vi "getStatusReport.vi"(2 "device":string, 3 "ListRef":refnum<queue>) -> (0 "output report":string)   [LabVIEW 2012]
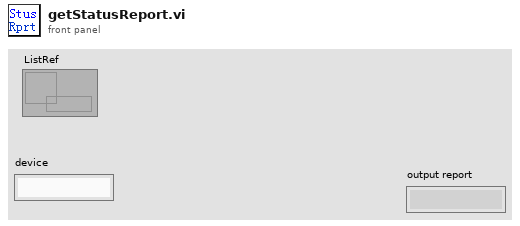
[diagram p1: front panel]
types:
  T1 = cluster{"DeviceID":string, "Channel":string, "param1":dbl, "Operation":string}
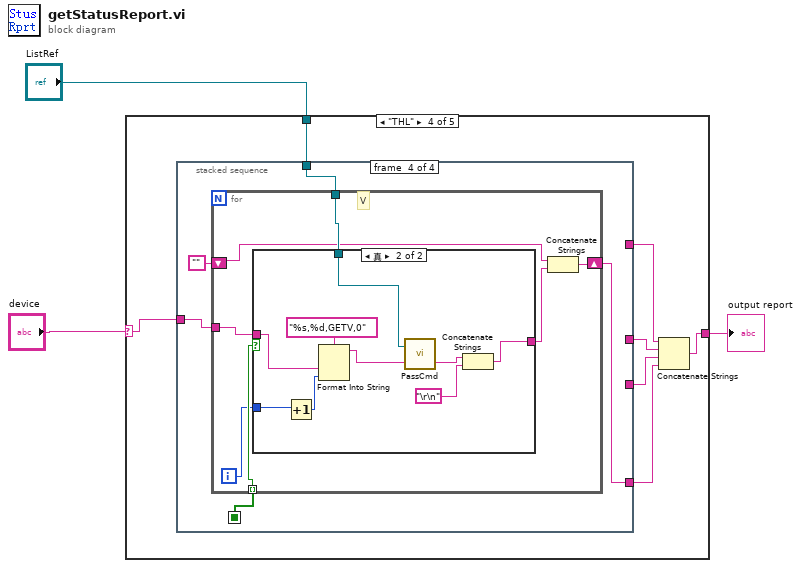
[diagram p0: block diagram]
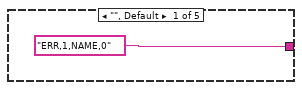
[diagram p2: hidden frame]
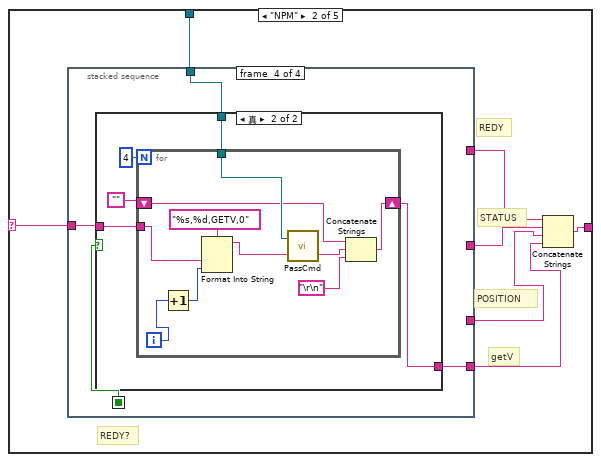
[diagram p3: hidden frame]
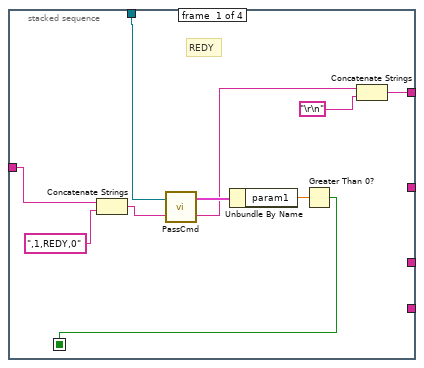
[diagram p4: hidden frame]
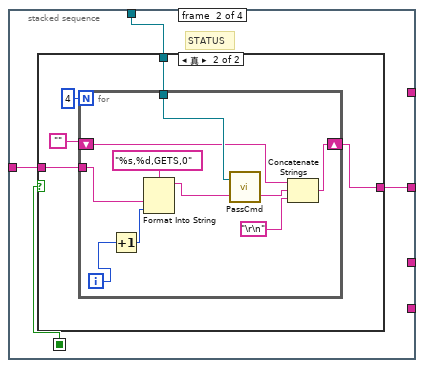
[diagram p5: hidden frame]
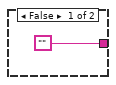
[diagram p6: hidden frame]
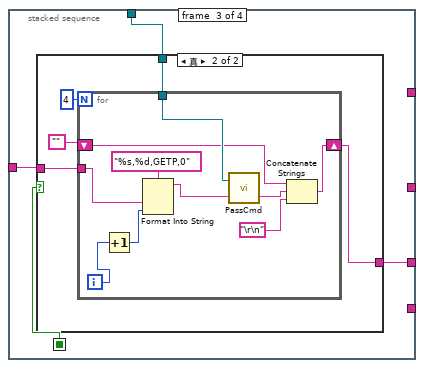
[diagram p7: hidden frame]
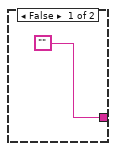
[diagram p8: hidden frame]
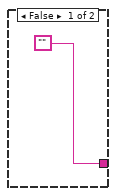
[diagram p9: hidden frame]
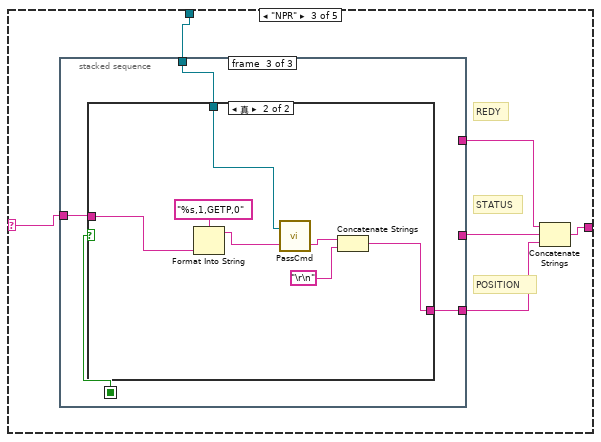
[diagram p10: hidden frame]
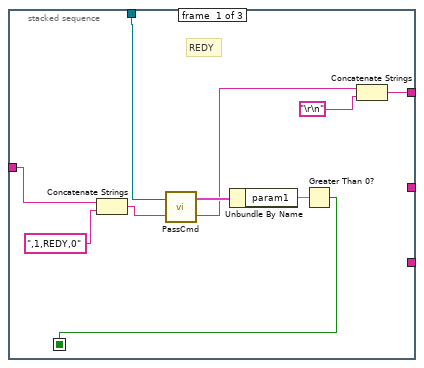
[diagram p11: hidden frame]
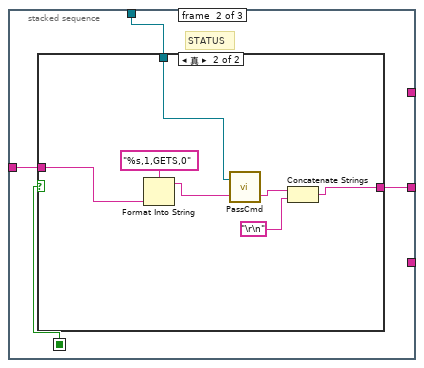
[diagram p12: hidden frame]
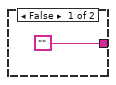
[diagram p13: hidden frame]
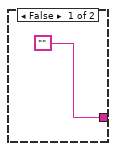
[diagram p14: hidden frame]
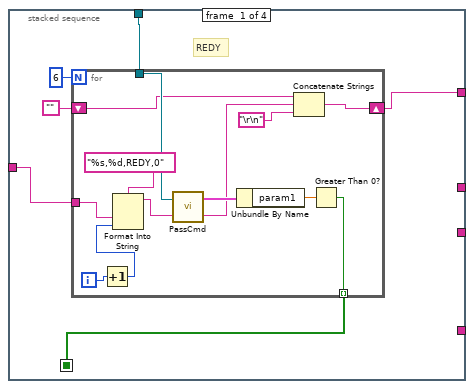
[diagram p15: hidden frame]
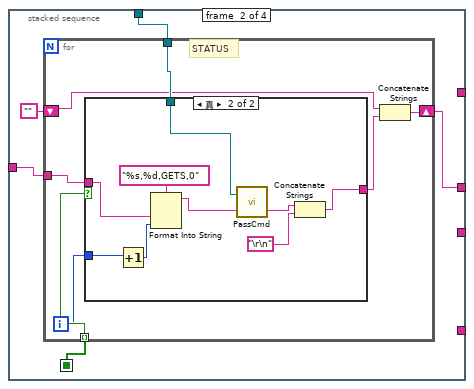
[diagram p16: hidden frame]
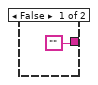
[diagram p17: hidden frame]
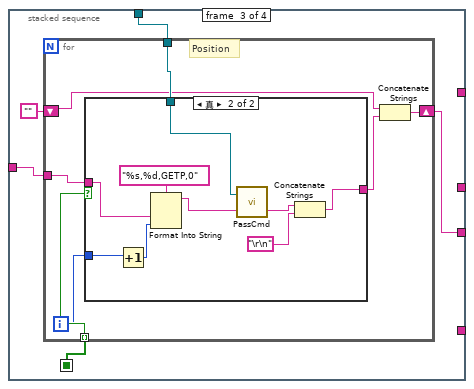
[diagram p18: hidden frame]
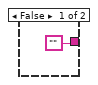
[diagram p19: hidden frame]
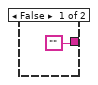
[diagram p20: hidden frame]
diagram:
  n1 = case shown="\"THL\"" "device" {
    selector: "device" -> [_ w11 w86 w127 w215]
    tunnel: ["ERR,1,NAME,0" w9 w82 w126 w214] -> w2
    tunnel: "ListRef" -> [_ w10 w87 w128 w216]
    frame "", Default {
    }
    frame "NPM" {
      # "getV"
      # "POSITION"
      # "STATUS"
      # "REDY"
      # "REDY?"
      n2 = stacked-sequence {
        seq-local: [w15 _ _ _] -> [_ w25 w45 w65]
        tunnel: w11 -> [w21 w24 w43 w63]
        tunnel: w10 -> [w18 w22 w44 w64]
        tunnel: [_ w23 _ _] -> w7
        tunnel: [w14 _ _ _] -> w8
        tunnel: [_ _ w42 _] -> w6
        tunnel: [_ _ _ w62] -> w5
        frame #0 {
          # "REDY"
          n3 = Concatenate Strings(w21, ",1,REDY,0") -> (w19:string)
          n4 = call "PassCmd.vi"("cmd in"=w19, "list ref"=w18) -> ("str out"=w13:string, "cmd out"=w17:T1)
          n5 = Unbundle By Name(w17) -> ("param1"=w16:dbl)
          n6 = Greater Than 0?(x=w16) -> (x > 0?=w15:bool)
          n7 = Concatenate Strings(w13, "\r\n") -> (w14:string)
        }
        frame #1 {
          # "STATUS"
          n8 = case shown="真" w25 {
            tunnel: w24 -> [_ w30]
            tunnel: ["" w27] -> w23
            tunnel: w22 -> [_ w29]
            frame False {
            }
            frame True {
              n9 = for {
                N: 4 -> [_]
                tunnel: w30 -> [w40]
                tunnel: w29 -> [w37]
                shift-right: [w33] -> w27
                shift-left: "" -> [w36]
                i -> [w32]
                n10 = Increment(x=w32) -> (x+1=w39:i32)
                n11 = Format Into String(format string="%s,%d,GETS,0" ("格式字符串"), w40, w39) -> (resulting string=w38:string)  [unwired: 2 in, 1 out]
                n12 = call "PassCmd.vi"("cmd in"=w38, "list ref"=w37) -> ("str out"=w35:string)  [unwired: 1 out]
                n13 = Concatenate Strings(w36, w35, "\r\n") -> (w33:string)
              }
            }
          }
        }
        frame #2 {
          n14 = case shown="真" w45 {
            tunnel: w43 -> [_ w50]
            tunnel: ["" w47] -> w42
            tunnel: w44 -> [_ w49]
            frame False {
            }
            frame True {
              n15 = for {
                N: 4 -> [_]
                tunnel: w50 -> [w60]
                tunnel: w49 -> [w57]
                shift-right: [w53] -> w47
                shift-left: "" -> [w56]
                i -> [w52]
                n16 = Increment(x=w52) -> (x+1=w59:i32)
                n17 = Format Into String(format string="%s,%d,GETP,0" ("格式字符串"), w60, w59) -> (resulting string=w58:string)  [unwired: 2 in, 1 out]
                n18 = call "PassCmd.vi"("cmd in"=w58, "list ref"=w57) -> ("str out"=w55:string)  [unwired: 1 out]
                n19 = Concatenate Strings(w56, w55, "\r\n") -> (w53:string)
              }
            }
          }
        }
        frame #3 {
          n20 = case shown="真" w65 {
            tunnel: w63 -> [_ w70]
            tunnel: ["" w67] -> w62
            tunnel: w64 -> [_ w69]
            frame False {
            }
            frame True {
              n21 = for {
                N: 4 -> [_]
                tunnel: w70 -> [w80]
                tunnel: w69 -> [w77]
                shift-right: [w73] -> w67
                shift-left: "" -> [w76]
                i -> [w72]
                n22 = Increment(x=w72) -> (x+1=w79:i32)
                n23 = Format Into String(format string="%s,%d,GETV,0" ("格式字符串"), w80, w79) -> (resulting string=w78:string)  [unwired: 2 in, 1 out]
                n24 = call "PassCmd.vi"("cmd in"=w78, "list ref"=w77) -> ("str out"=w75:string)  [unwired: 1 out]
                n25 = Concatenate Strings(w76, w75, "\r\n") -> (w73:string)
              }
            }
          }
        }
      }
      n26 = Concatenate Strings(w8, w7, w6, w5) -> (w9:string)
    }
    frame "NPR" {
      # "POSITION"
      # "STATUS"
      # "REDY"
      n27 = stacked-sequence {
        seq-local: [w91 _ _] -> [_ w101 w113]
        tunnel: w86 -> [w97 w100 w111]
        tunnel: w87 -> [w94 w98 w112]
        tunnel: [_ w99 _] -> w84
        tunnel: [w90 _ _] -> w85
        tunnel: [_ _ w110] -> w83
        frame #0 {
          # "REDY"
          n28 = Concatenate Strings(w97, ",1,REDY,0") -> (w95:string)
          n29 = call "PassCmd.vi"("cmd in"=w95, "list ref"=w94) -> ("str out"=w89:string, "cmd out"=w93:T1)
          n30 = Unbundle By Name(w93) -> ("param1"=w92:dbl)
          n31 = Greater Than 0?(x=w92) -> (x > 0?=w91:bool)
          n32 = Concatenate Strings(w89, "\r\n") -> (w90:string)
        }
        frame #1 {
          # "STATUS"
          n33 = case shown="真" w101 {
            tunnel: w100 -> [_ w109]
            tunnel: ["" w107] -> w99
            tunnel: w98 -> [_ w108]
            frame False {
            }
            frame True {
              n34 = Format Into String(format string="%s,1,GETS,0" ("格式字符串"), w109) -> (resulting string=w105:string)  [unwired: 2 in, 1 out]
              n35 = call "PassCmd.vi"("cmd in"=w105, "list ref"=w108) -> ("str out"=w104:string)  [unwired: 1 out]
              n36 = Concatenate Strings(w104, "\r\n") -> (w107:string)
            }
          }
        }
        frame #2 {
          n37 = case shown="真" w113 {
            tunnel: w111 -> [_ w121]
            tunnel: ["" w119] -> w110
            tunnel: w112 -> [_ w120]
            frame False {
            }
            frame True {
              n38 = Format Into String(format string="%s,1,GETP,0" ("格式字符串"), w121) -> (resulting string=w117:string)  [unwired: 2 in, 1 out]
              n39 = call "PassCmd.vi"("cmd in"=w117, "list ref"=w120) -> ("str out"=w116:string)  [unwired: 1 out]
              n40 = Concatenate Strings(w116, "\r\n") -> (w119:string)
            }
          }
        }
      }
      n41 = Concatenate Strings(w85, w84, w83) -> (w82:string)
    }
    frame "THL" {
      n42 = stacked-sequence {
        seq-local: [w132 _ _ _] -> [_ w149 w172 w194]
        tunnel: w127 -> [w134 w152 w174 w196]
        tunnel: w128 -> [w133 w150 w173 w195]
        tunnel: [_ w151 _ _] -> w124
        tunnel: [w131 _ _ _] -> w125
        tunnel: [_ _ w170 _] -> w123
        tunnel: [_ _ _ w192] -> w122
        frame #0 {
          # "REDY"
          n43 = for {
            N: 6 -> [_]
            tunnel: w134 -> [w137]
            tunnel: w133 -> [w147]
            tunnel: [w144] -> w132 mode=indexing
            shift-right: [w143] -> w131
            shift-left: "" -> [w136]
            i -> [w139]
            n44 = Increment(x=w139) -> (x+1=w138:i32)
            n45 = Format Into String(format string="%s,%d,REDY,0", w137, w138) -> (resulting string=w135:string)  [unwired: 2 in, 1 out]
            n46 = call "PassCmd.vi"("cmd in"=w135, "list ref"=w147) -> ("str out"=w142:string, "cmd out"=w146:T1)
            n47 = Unbundle By Name(w146) -> ("param1"=w145:dbl)
            n48 = Concatenate Strings(w136, w142, "\r\n") -> (w143:string)
            n49 = Greater Than 0?(x=w145) -> (x > 0?=w144:bool)
          }
        }
        frame #1 {
          n50 = for {
            tunnel: w152 -> [w159]
            tunnel: w150 -> [w158]
            tunnel: w149 -> [w157] mode=indexing
            shift-right: [w155] -> w151
            shift-left: "" -> [w153]
            i -> [w156]
            # "STATUS"
            n51 = case shown="真" w157 {
              tunnel: w159 -> [_ w169]
              tunnel: ["" w168] -> w154
              tunnel: w158 -> [_ w167]
              tunnel: w156 -> [_ w161]
              frame False {
              }
              frame True {
                n52 = Increment(x=w161) -> (x+1=w165:i32)
                n53 = Format Into String(format string="%s,%d,GETS,0" ("格式字符串"), w169, w165) -> (resulting string=w164:string)  [unwired: 2 in, 1 out]
                n54 = call "PassCmd.vi"("cmd in"=w164, "list ref"=w167) -> ("str out"=w163:string)  [unwired: 1 out]
                n55 = Concatenate Strings(w163, "\r\n") -> (w168:string)
              }
            }
            n56 = Concatenate Strings(w153, w154) -> (w155:string)
          }
        }
        frame #2 {
          n57 = for {
            tunnel: w174 -> [w181]
            tunnel: w173 -> [w180]
            tunnel: w172 -> [w179] mode=indexing
            shift-right: [w177] -> w170
            shift-left: "" -> [w175]
            i -> [w178]
            # "Position"
            n58 = case shown="真" w179 {
              tunnel: w181 -> [_ w191]
              tunnel: ["" w190] -> w176
              tunnel: w180 -> [_ w189]
              tunnel: w178 -> [_ w183]
              frame False {
              }
              frame True {
                n59 = Increment(x=w183) -> (x+1=w187:i32)
                n60 = Format Into String(format string="%s,%d,GETP,0" ("格式字符串"), w191, w187) -> (resulting string=w186:string)  [unwired: 2 in, 1 out]
                n61 = call "PassCmd.vi"("cmd in"=w186, "list ref"=w189) -> ("str out"=w185:string)  [unwired: 1 out]
                n62 = Concatenate Strings(w185, "\r\n") -> (w190:string)
              }
            }
            n63 = Concatenate Strings(w175, w176) -> (w177:string)
          }
        }
        frame #3 {
          n64 = for {
            tunnel: w196 -> [w203]
            tunnel: w195 -> [w202]
            tunnel: w194 -> [w201] mode=indexing
            shift-right: [w199] -> w192
            shift-left: "" -> [w197]
            i -> [w200]
            # "V"
            n65 = case shown="真" w201 {
              tunnel: w203 -> [_ w213]
              tunnel: ["" w212] -> w198
              tunnel: w202 -> [_ w211]
              tunnel: w200 -> [_ w205]
              frame False {
              }
              frame True {
                n66 = Increment(x=w205) -> (x+1=w209:i32)
                n67 = Format Into String(format string="%s,%d,GETV,0" ("格式字符串"), w213, w209) -> (resulting string=w208:string)  [unwired: 2 in, 1 out]
                n68 = call "PassCmd.vi"("cmd in"=w208, "list ref"=w211) -> ("str out"=w207:string)  [unwired: 1 out]
                n69 = Concatenate Strings(w207, "\r\n") -> (w212:string)
              }
            }
            n70 = Concatenate Strings(w197, w198) -> (w199:string)
          }
        }
      }
      n71 = Concatenate Strings(w125, w124, w123, w122) -> (w126:string)
    }
    frame "PIZ" {
      # "POSITION"
      # "STATUS"
      # "REDY"
      n72 = stacked-sequence {
        seq-local: [w223 _ _] -> [_ w233 w245]
        tunnel: w215 -> [w229 w232 w243]
        tunnel: w216 -> [w226 w230 w244]
        tunnel: [_ w231 _] -> w218
        tunnel: [w222 _ _] -> w217
        tunnel: [_ _ w242] -> w219
        frame #0 {
          # "REDY"
          n73 = Concatenate Strings(w229, ",1,REDY,0") -> (w227:string)
          n74 = call "PassCmd.vi"("cmd in"=w227, "list ref"=w226) -> ("str out"=w221:string, "cmd out"=w225:T1)
          n75 = Unbundle By Name(w225) -> ("param1"=w224:dbl)
          n76 = Greater Than 0?(x=w224) -> (x > 0?=w223:bool)
          n77 = Concatenate Strings(w221, "\r\n") -> (w222:string)
        }
        frame #1 {
          # "STATUS"
          n78 = case shown="真" w233 {
            tunnel: w232 -> [_ w241]
            tunnel: ["" w239] -> w231
            tunnel: w230 -> [_ w240]
            frame False {
            }
            frame True {
              n79 = Format Into String(format string="%s,1,GETS,0" ("格式字符串"), w241) -> (resulting string=w237:string)  [unwired: 2 in, 1 out]
              n80 = call "PassCmd.vi"("cmd in"=w237, "list ref"=w240) -> ("str out"=w236:string)  [unwired: 1 out]
              n81 = Concatenate Strings(w236, "\r\n") -> (w239:string)
            }
          }
        }
        frame #2 {
          n82 = case shown="真" w245 {
            tunnel: w243 -> [_ w253]
            tunnel: ["" w251] -> w242
            tunnel: w244 -> [_ w252]
            frame False {
            }
            frame True {
              n83 = Format Into String(format string="%s,1,GETP,0" ("格式字符串"), w253) -> (resulting string=w249:string)  [unwired: 2 in, 1 out]
              n84 = call "PassCmd.vi"("cmd in"=w249, "list ref"=w252) -> ("str out"=w248:string)  [unwired: 1 out]
              n85 = Concatenate Strings(w248, "\r\n") -> (w251:string)
            }
          }
        }
      }
      n86 = Concatenate Strings(w217, w218, w219) -> (w214:string)
    }
  }
  "output report" <- w2
